vi "HW_GEN - Get Display Data from Queue.vi"(7 "Time Out(-1)":i32, 8 "error in":errorcluster, 11 "Object Name":string) -> (0 "error out":errorcluster, 2 "data":waveform(dbl)[](array[waveform]), 3 "Object Name Out":string)   [LabVIEW 2016]
doc: "从数据队列中获取数据用于显示"
uses:
  Ctrls/HardWare _ Queue Data Type.ctl
panel:
  # "Data Out"
  # "Data In"
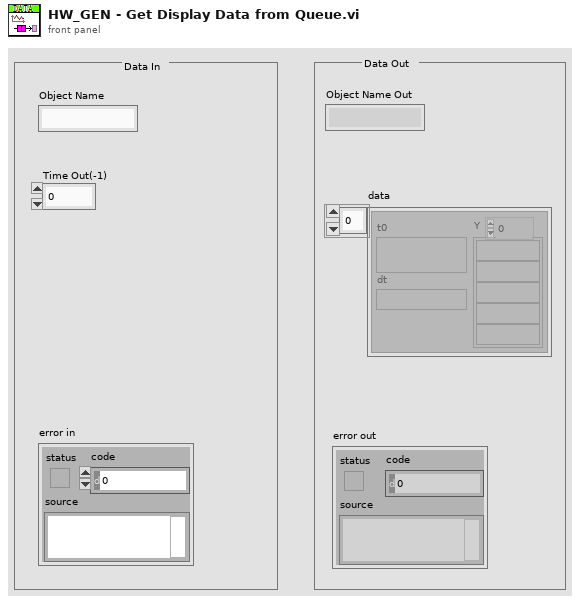
[diagram p1: front panel]
types:
  T1 = typedef "HardWare _ Queue Data Type.ctl" = cluster{"UnitNo.":i32, "data":dbl[][], "T0":dbl, "SampRate":dbl}
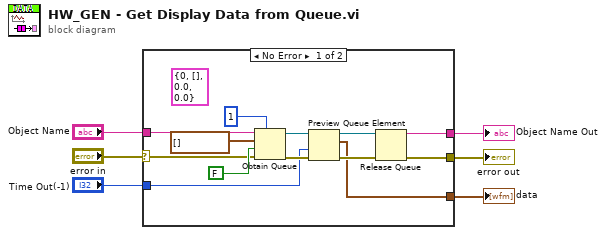
[diagram p0: block diagram]
diagram:
  n1 = case shown="No Error" "error in" {
    selector: "error in" -> [w14 w21]
    tunnel: [w17 w21] -> w6
    tunnel: "Object Name" -> [w16 w20]
    tunnel: [w10 _] -> w2
    tunnel: [w9 w20] -> w3
    tunnel: "Time Out(-1)" -> [w8 _]
    frame No Error {
      (unwired) T1 {"UnitNo."=0, "data"=[], "T0"=0.0, "SampRate"=0.0} ("Wave")
      n2 = Obtain Queue(max queue size (-1, unlimited)=1 ("队列最大值（-1，无限）"), name (unnamed)=w16, element data type=waveform(dbl)[] [] ("data"), create if not found? (T)=FALSE ("如未找到是否创建？(T)"), error in (no error)=w14) -> (queue out=w18:refnum<queue>, error out=w12:errorcluster)  [unwired: 1 out]
      n3 = Preview Queue Element(queue=w18, timeout in ms (-1)=w8, error in (no error)=w12) -> (queue out=w13:refnum<queue>, element=w10:waveform(dbl)[], error out=w11:errorcluster)  [unwired: 1 out]
      n4 = Release Queue(queue=w13, error in (no error)=w11) -> (queue name=w9:string, error out=w17:errorcluster)  [unwired: 1 in, 1 out]
    }
    frame Error {
    }
  }
  "error out" <- w6
  "Object Name Out" <- w3
  "data" <- w2
